vi "OPCUAServer.vi"() -> ()   [LabVIEW 2018]
uses:
  <vilib>/OPCUA/server/Read Double.vi
  <vilib>/OPCUA/NI OPC UA Server.lvlib
panel:
  in  "Tab Control":enum32{"OPC", "SQL Server", "Error Handler"}(tab)
  out "Temperature [C]":dbl=25.00772115553251 format="%.2g"
  out "Server Endpoint URL":string="opc.tcp://XPS15HPH:49580"
  out "Item Node Id":string="ns=2;s=ProcessData.Temperature"
  in  "Write to SQL Server":bool
  in  "Database Connection":T1={"Data Source Name"="XPS15HPH\\SQLEXPRESS", "Database Name"="MEASUREMENTS", "User Name"="sa", "Password"="ullabella"}
  out "Error Message":errorcluster
  out "Status":bool
  out "Current Time":string="2018-10-12 13:39:17"
  out "Error Out":errorcluster
  in  "Error In":errorcluster
  in  "Stop OPC Server":bool
  in  "Start OPC Server":bool
  in  "Exit Button":bool
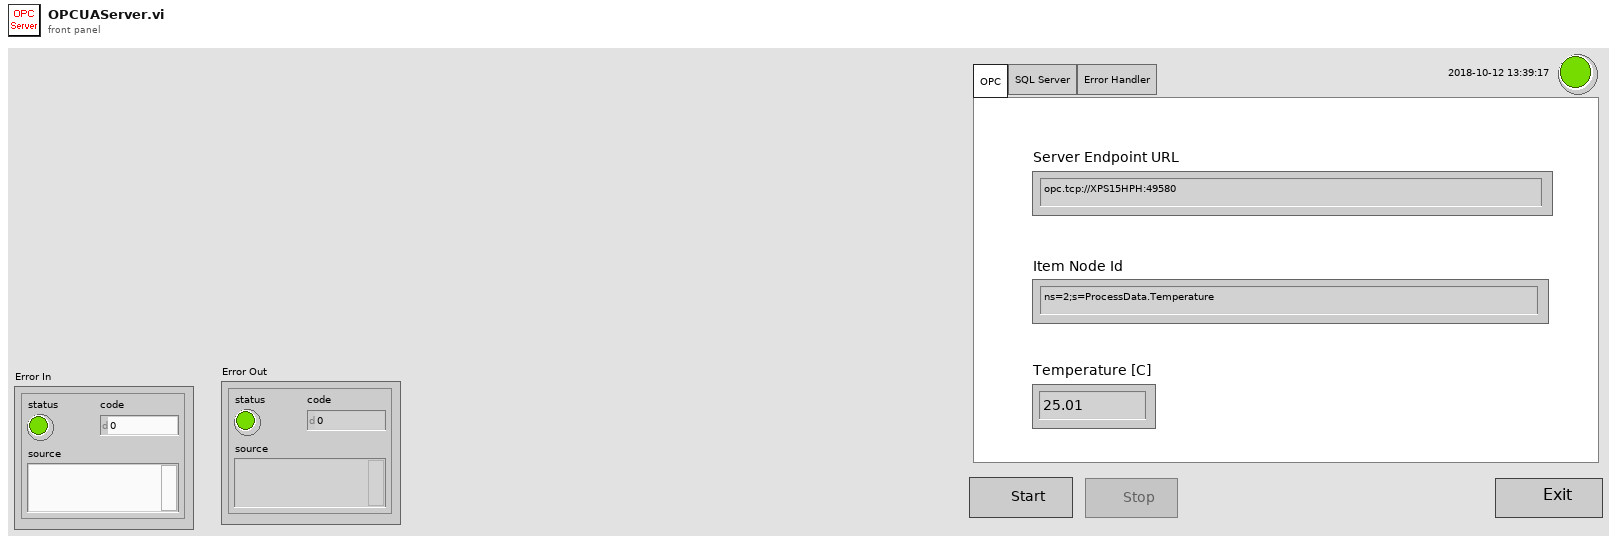
[diagram p1: front panel]
types:
  T1 = cluster{"Data Source Name":string, "Database Name":string, "User Name":string, "Password":string}
  T2 = enum8{"Enabled", "Disabled", "Disabled and Grayed Out"}
  T3 = cluster{"name":string, "data type":u16, "access level":u16, "description":string}
  T4 = typedef "OPC UA Server Refnum.ctl" = refnum<k21>
  T5 = typedef "NodeId.ctl" = string
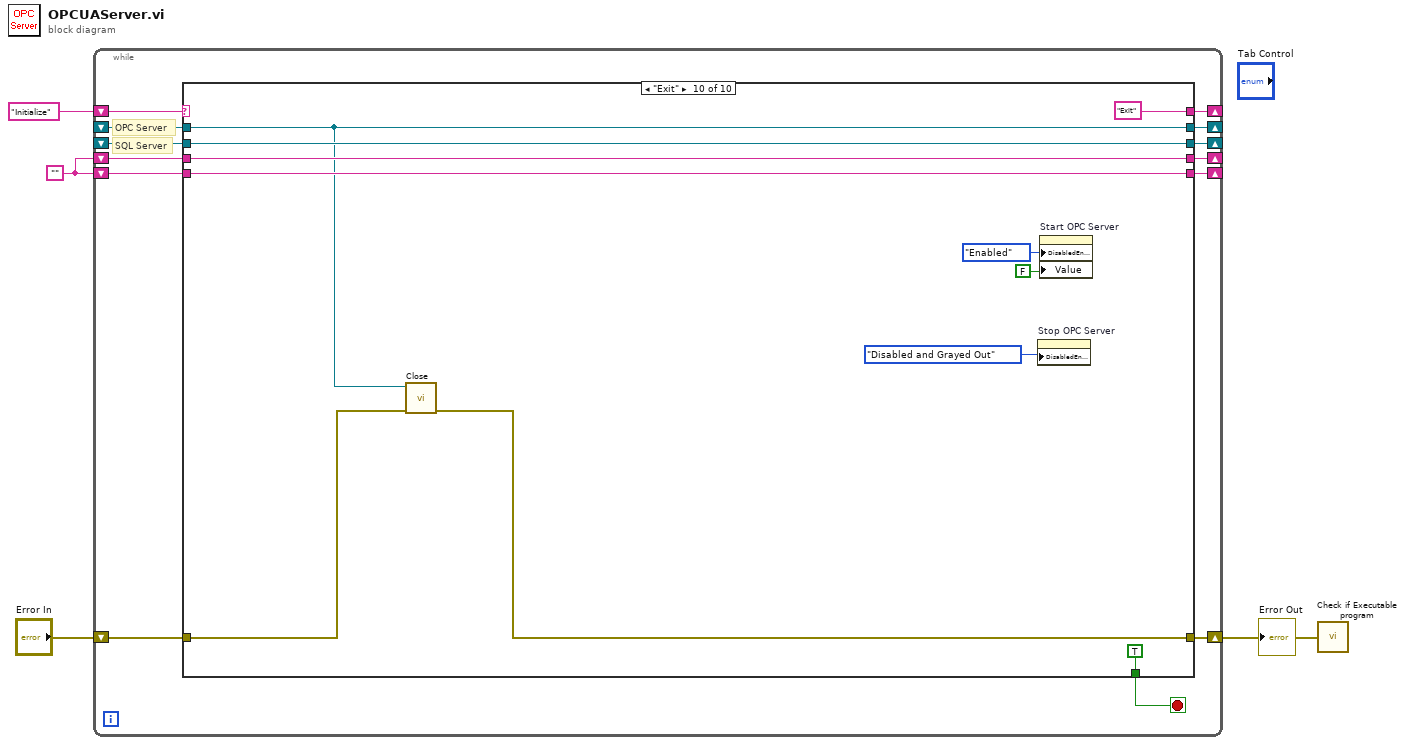
[diagram p0: block diagram]
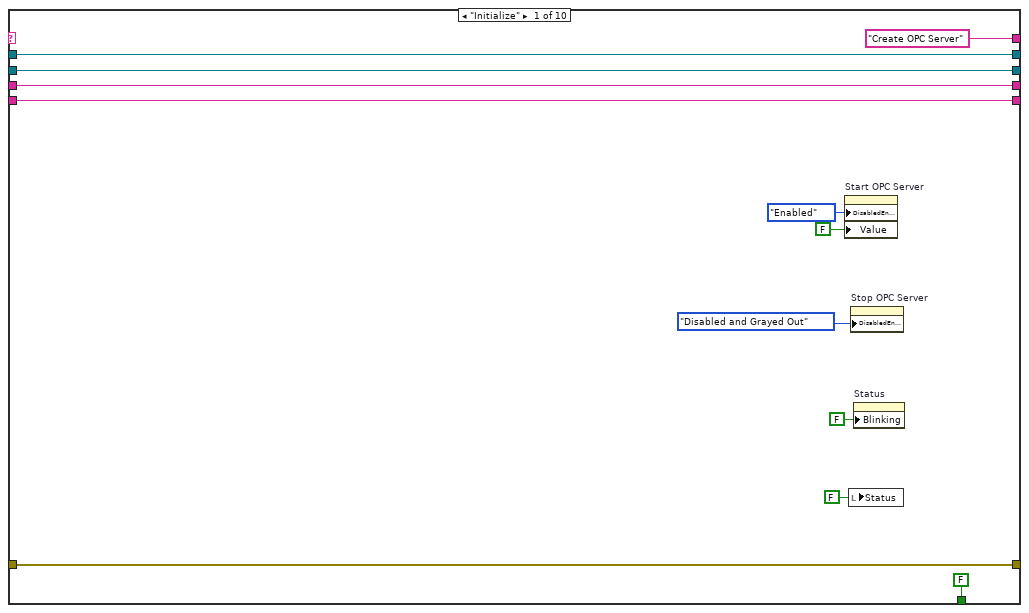
[diagram p2: hidden frame]
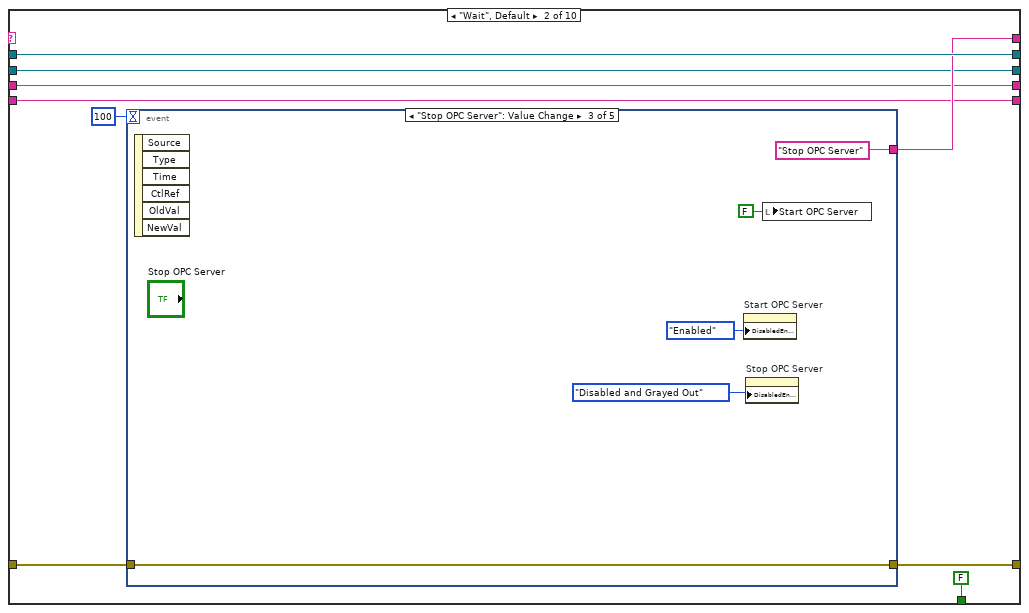
[diagram p3: hidden frame]
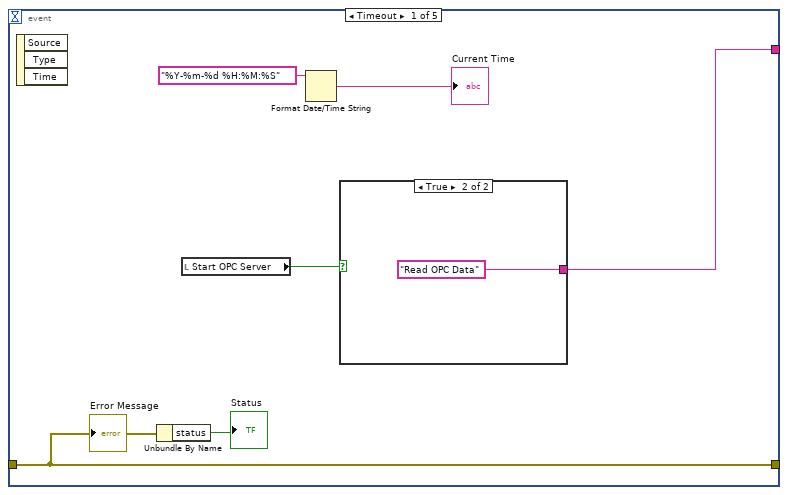
[diagram p4: hidden frame]
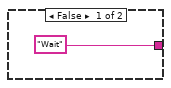
[diagram p5: hidden frame]
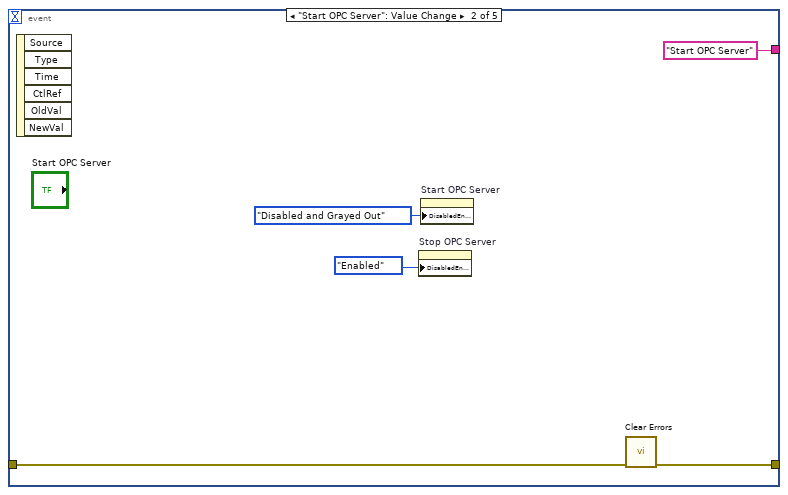
[diagram p6: hidden frame]
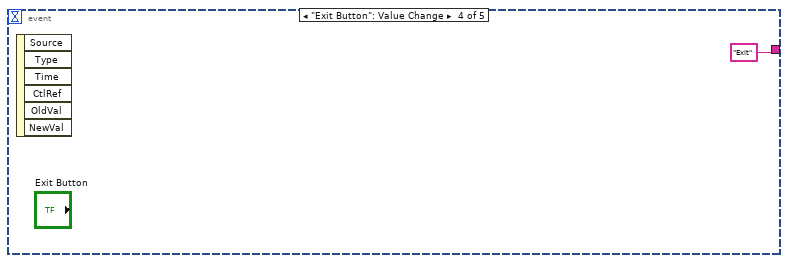
[diagram p7: hidden frame]
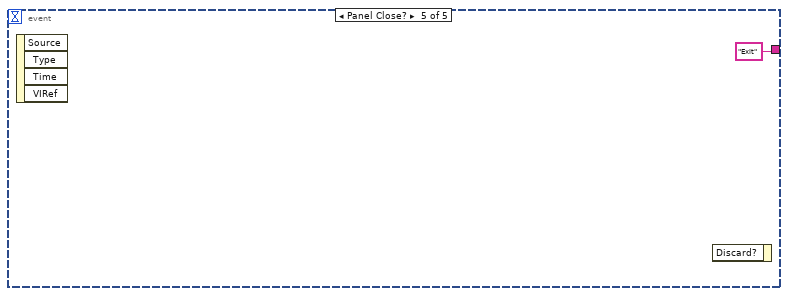
[diagram p8: hidden frame]
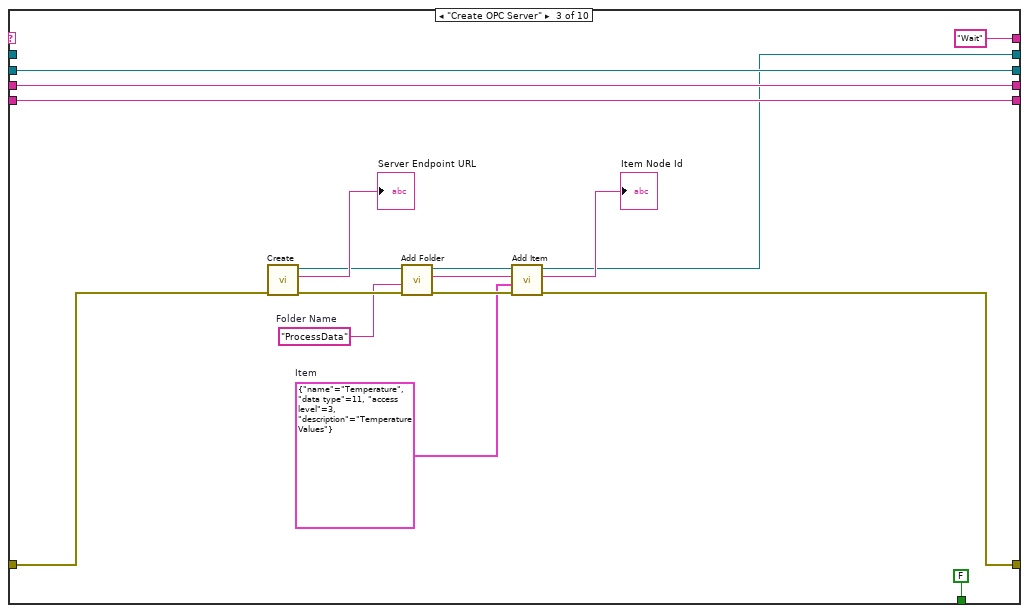
[diagram p9: hidden frame]
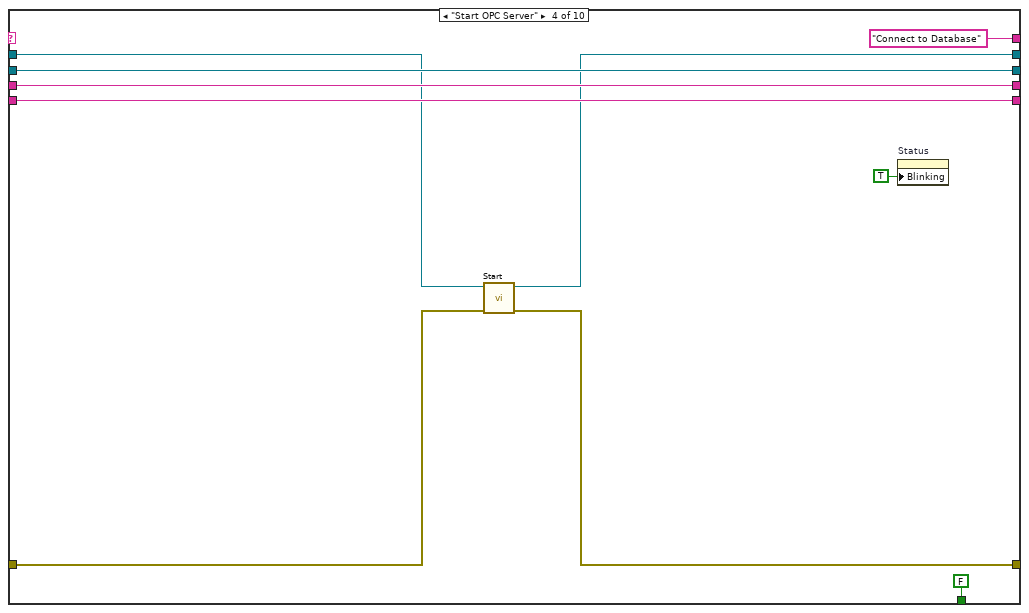
[diagram p10: hidden frame]
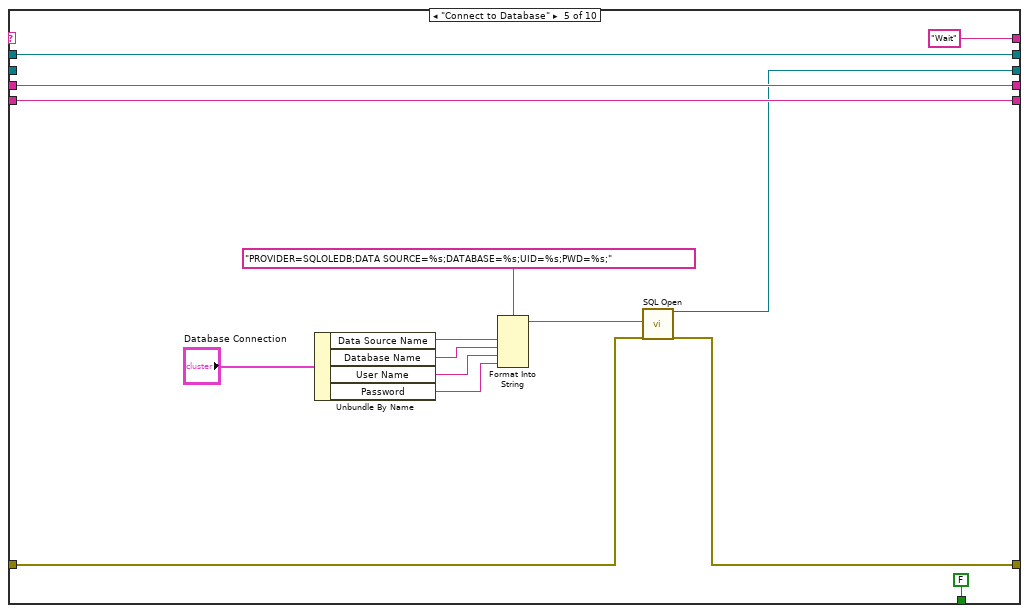
[diagram p11: hidden frame]
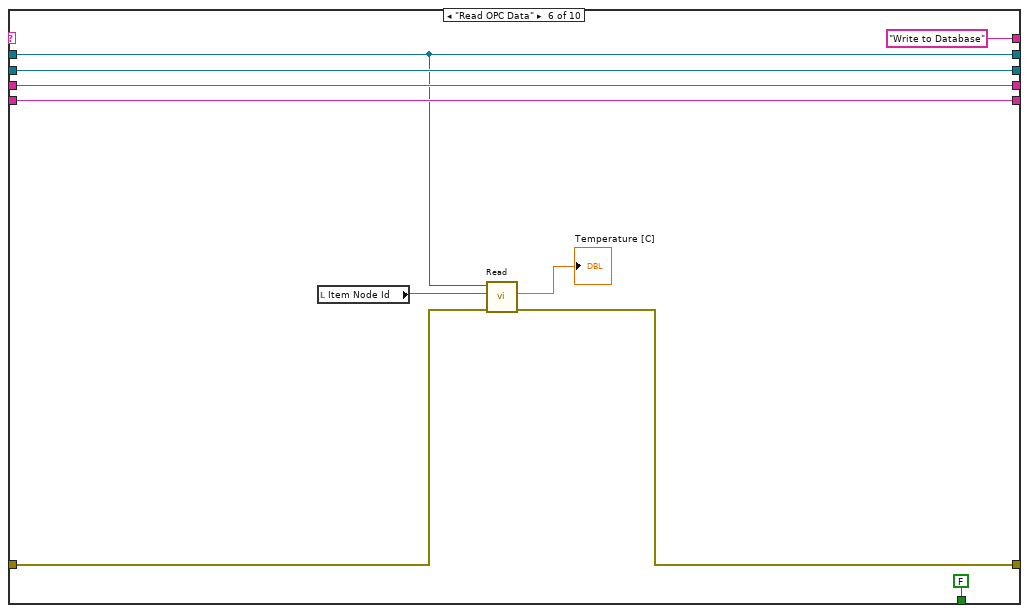
[diagram p12: hidden frame]
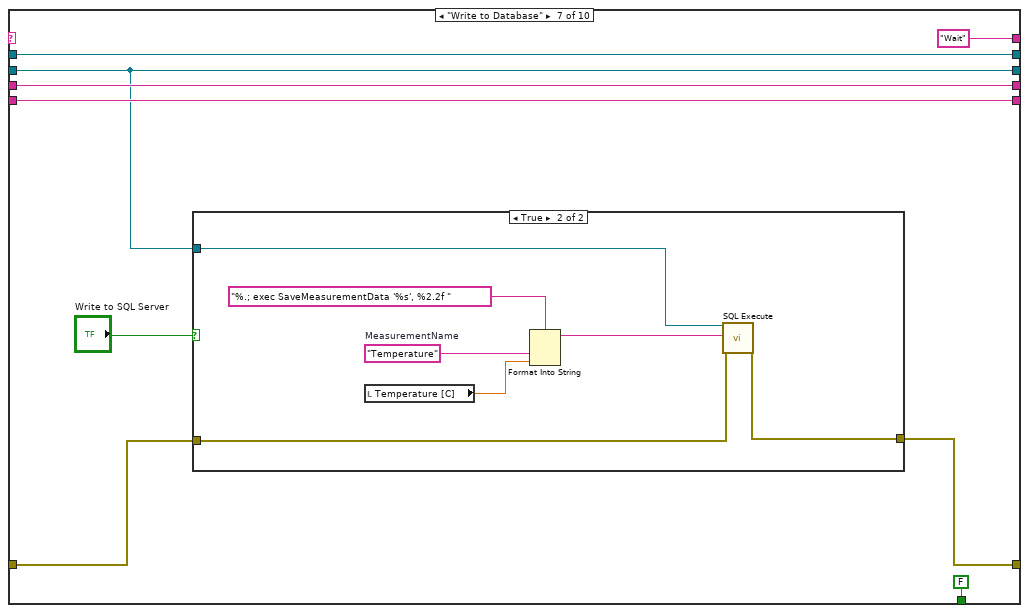
[diagram p13: hidden frame]
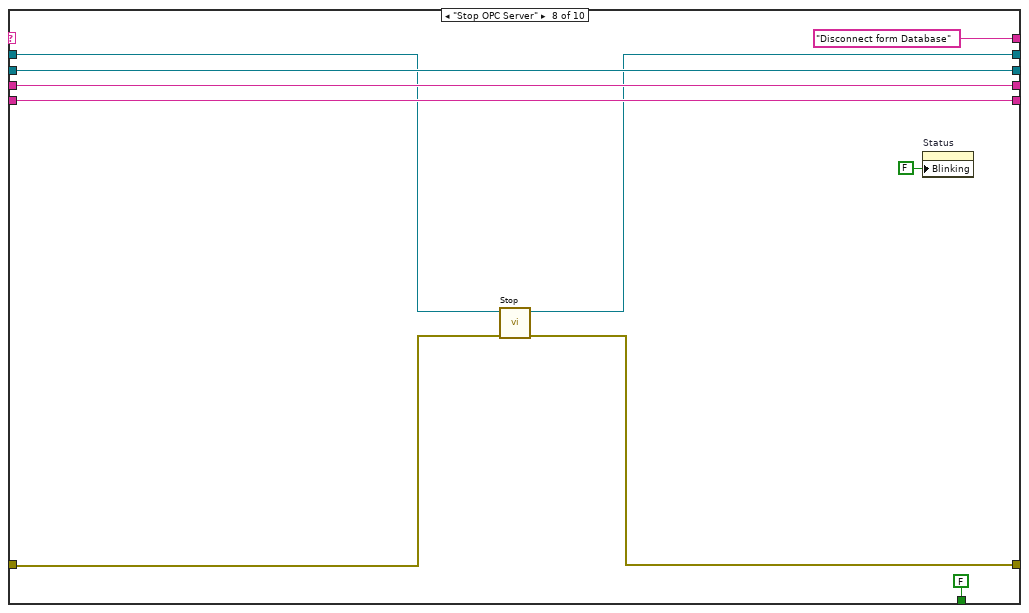
[diagram p15: hidden frame]
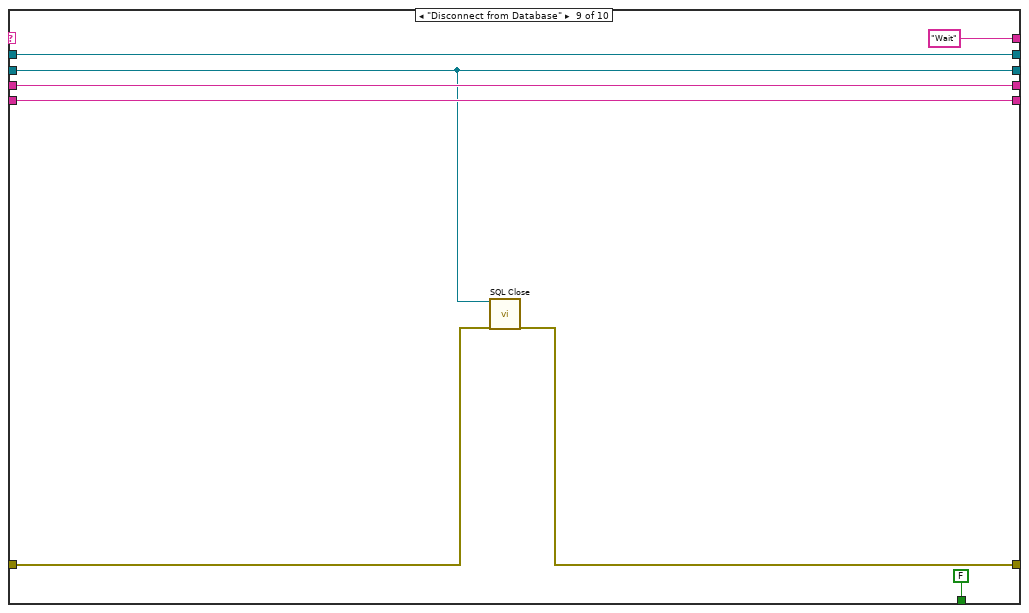
[diagram p16: hidden frame]
diagram:
  w2 = ""
  n1 = while {
    shift-right: [w16] -> _
    shift-left: "Initialize" -> [w17]
    shift-right: [w14] -> _
    shift-left: _ -> [w15]
    shift-right: [w11] -> _
    shift-left: _ -> [w12]
    shift-right: [w9] -> _
    shift-left: w2 -> [w10]
    shift-right: [w7] -> _
    shift-left: w2 -> [w8]
    shift-right: [w5] -> w1
    shift-left: "Error In" -> [w6]
    stop <- w13 stop-if-true
    # "SQL Server"
    # "OPC Server"
    n2 = case shown="\"Exit\"" w17 {
      tunnel: ["Create OPC Server" w36 "Wait" "Connect to Database" "Wait" "Write to Database" "Wait" "Disconnect form Database" "Wait" "Exit"] -> w16
      tunnel: w15 -> [w28 w37 _ w77 w100 w105 w119 w131 w145 w148]
      tunnel: [w28 w37 w60 w78 w100 w105 w119 w132 w145 w148] -> w14
      tunnel: [FALSE FALSE FALSE FALSE FALSE FALSE FALSE FALSE FALSE TRUE] -> w13
      tunnel: w12 -> [w26 w34 w71 w84 _ w109 w111 w133 w138 w155]
      tunnel: [w26 w34 w71 w84 w86 w109 w111 w133 w138 w155] -> w11
      tunnel: w10 -> [w25 w33 w74 w83 w98 w108 w116 w136 w143 w154]
      tunnel: [w25 w33 w74 w83 w98 w108 w116 w136 w143 w154] -> w9
      tunnel: w8 -> [w24 w32 w73 w82 w97 w107 w115 w135 w142 w153]
      tunnel: [w24 w32 w73 w82 w97 w107 w115 w135 w142 w153] -> w7
      tunnel: w6 -> [w23 w30 w61 w79 w95 w103 w114 w130 w140 w146]
      tunnel: [w23 w31 w59 w80 w94 w104 w113 w129 w139 w147] -> w5
      frame "Initialize" {
        n3 = property on="Start OPC Server" class="Bool (strict)"("DisabledEnum"=T2."Enabled" ("Disabled"), "Value"=FALSE ("Start DAQ Button")) -> ()  [unwired: 2 in, 2 out]
        n4 = local write "Status"(FALSE ("Status")) -> ()
        n5 = property on="Stop OPC Server" class="Bool"("DisabledEnum"=T2."Disabled and Grayed Out" ("Disabled")) -> ()  [unwired: 2 in, 2 out]
        n6 = property on="Status" class="Bool (strict)"("Blinking"=FALSE) -> ()  [unwired: 2 in, 2 out]
      }
      frame "Wait", Default {
        n7 = event shown="[2] \"Stop OPC Server\": Value Change" {
          selector: _ -> [_ _ _ _ _]
          dyn-events: _ -> [_ _ _ _ _]
          timeout: 100 -> [_ _ _ _ _]
          tunnel: [w41 "Start OPC Server" "Stop OPC Server" "Exit" "Exit"] -> w36
          tunnel: w30 -> [w39 w48 w56 _ _]
          tunnel: [w39 w47 w56 _ _] -> w31
          event Timeout {
            n8 = event-data() -> ()  [unwired: 1 in, 3 out]
            n9 = Unbundle By Name(w39) -> ("status"=→"Status":bool)
            n10 = local read "Start OPC Server"() -> (w42:bool)
            n11 = Format Date/Time String(time format string (%c)="%Y-%m-%d %H:%M:%S") -> (date/time string=→"Current Time":string)  [unwired: 2 in]
            n12 = case shown="True" w42 {
              tunnel: ["Wait" "Read OPC Data"] -> w41
              frame False {
              }
              frame True {
              }
            }
            "Error Message" <- w39
          }
          event "Start OPC Server": Value Change {
            n13 = event-data() -> ()  [unwired: 1 in, 6 out]
            n14 = property on="Stop OPC Server" class="Bool"("DisabledEnum"=T2."Enabled" ("Disabled")) -> ()  [unwired: 2 in, 2 out]
            n15 = property on="Start OPC Server" class="Bool (strict)"("DisabledEnum"=T2."Disabled and Grayed Out" ("Disabled")) -> ()  [unwired: 2 in, 2 out]
            n16 = call <vilib>:"Clear Errors.vi"("error in (no error)"=w48) -> ("error out"=w47:errorcluster)  [unwired: 5 in, 1 out]
          }
          event "Stop OPC Server": Value Change {
            n17 = event-data() -> ()  [unwired: 1 in, 6 out]
            n18 = property on="Start OPC Server" class="Bool (strict)"("DisabledEnum"=T2."Enabled" ("Disabled")) -> ()  [unwired: 2 in, 2 out]
            n19 = property on="Stop OPC Server" class="Bool"("DisabledEnum"=T2."Disabled and Grayed Out" ("Disabled")) -> ()  [unwired: 2 in, 2 out]
            n20 = local write "Start OPC Server"(FALSE ("Start OPC Server")) -> ()
          }
          event "Exit Button": Value Change {
            n21 = event-data() -> ()  [unwired: 1 in, 6 out]
          }
          event Panel Close? {
            n22 = event-data() -> ()  [unwired: 1 in, 4 out]
            n23 = event-data() -> ()  [unwired: 2 in, 1 out]
          }
        }
      }
      frame "Create OPC Server" {
        w63 = T3 {"name"="Temperature", "data type"=11, "access level"=3, "description"="Temperature Values"}  # Item
        w67 = "ProcessData"  # Folder Name
        n24 = call <vilib>:"Create.vi"("error in (no error)"=w61) -> ("error out"=w70:errorcluster, "server endpoint URL"=→"Server Endpoint URL":string, "OPC UA server refnum out"=w66:T4)  [unwired: 8 in]
        n25 = call <vilib>:"Add Folder.vi"("error in (no error)"=w70, "folder name"=w67, "OPC UA server refnum in"=w66) -> ("error out"=w69:errorcluster, "folder node ID"=w64:T5, "OPC UA server refnum out"=w65:T4)  [unwired: 5 in]
        n26 = call <vilib>:"Add Item.vi"("error in (no error)"=w69, "item"=w63, "parent folder node ID"=w64, "OPC UA server refnum in"=w65) -> ("error out"=w59:errorcluster, "item node ID"=→"Item Node Id":T5, "OPC UA server refnum out"=w60:T4)  [unwired: 3 in, 1 out]
      }
      frame "Start OPC Server" {
        n27 = call <vilib>:"Start.vi"("error in (no error)"=w79, "OPC UA server refnum in"=w77) -> ("error out"=w80:errorcluster, "OPC UA server refnum out"=w78:T4)  [unwired: 7 in, 1 out]
        n28 = property on="Status" class="Bool (strict)"("Blinking"=TRUE) -> ()  [unwired: 2 in, 2 out]
      }
      frame "Connect to Database" {
        n29 = Unbundle By Name("Database Connection") -> ("Data Source Name"=w90:string, "Database Name"=w89:string, "User Name"=w88:string, "Password"=w87:string)
        n30 = Format Into String(format string="PROVIDER=SQLOLEDB;DATA SOURCE=%s;DATABASE=%s;UID=%s;PWD=%s;", w90, w89, w88, w87) -> (resulting string=w92:string)  [unwired: 2 in, 1 out]
        n31 = call <vilib>:"SQL Open.vi"("ConnectionString In"=w92, "Error in (no error)"=w95) -> ("Connection Out"=w86:refnum<k7>, "Error out"=w94:errorcluster)  [unwired: 16 in]
      }
      frame "Read OPC Data" {
        n32 = local read "Item Node Id"() -> (w102:string)
        n33 = call-poly <vilib>:"Read.vi"("error in (no error)"=w103, "node ID"=w102, "OPC UA server refnum in"=w105) -> ("error out"=w104:errorcluster, "value"=→"Temperature [C]":dbl)  [unwired: 4 in, 3 out]
      }
      frame "Write to Database" {
        n34 = case shown="True" "Write to SQL Server" {
          tunnel: w114 -> [w120 w123]
          tunnel: [w120 w122] -> w113
          tunnel: w111 -> [_ w121]
          frame False {
          }
          frame True {
            w125 = "Temperature"  # MeasurementName
            n35 = local read "Temperature [C]"() -> (w124:dbl)
            n36 = Format Into String "Format Into String"(format string="%.; exec SaveMeasurementData '%s', %2.2f ", w125, w124) -> (resulting string=w126:string)  [unwired: 2 in, 1 out]
            n37 = call <vilib>:"SQL Execute.vi"("Connection In"=w121, "SQL Query"=w126, "Error in (no error)"=w123) -> ("Error out"=w122:errorcluster)  [unwired: 15 in, 1 out]
          }
        }
      }
      frame "Stop OPC Server" {
        n38 = call <vilib>:"Stop.vi"("error in (no error)"=w130, "OPC UA server refnum in"=w131) -> ("error out"=w129:errorcluster, "OPC UA server refnum out"=w132:T4)  [unwired: 8 in]
        n39 = property on="Status" class="Bool (strict)"("Blinking"=FALSE) -> ()  [unwired: 2 in, 2 out]
      }
      frame "Disconnect from Database" {
        n40 = call <vilib>:"SQL Close.vi"("Connection In"=w138, "Error in (no error)"=w140) -> ("Error out"=w139:errorcluster)  [unwired: 17 in]
      }
      frame "Exit" {
        n41 = call <vilib>:"Close.vi"("error in (no error)"=w146, "OPC UA server refnum in"=w148) -> ("error out"=w147:errorcluster)  [unwired: 9 in]
        n42 = property on="Stop OPC Server" class="Bool"("DisabledEnum"=T2."Disabled and Grayed Out" ("Disabled")) -> ()  [unwired: 2 in, 2 out]
        n43 = property on="Start OPC Server" class="Bool (strict)"("DisabledEnum"=T2."Enabled" ("Disabled"), "Value"=FALSE ("Start DAQ Button")) -> ()  [unwired: 2 in, 2 out]
      }
    }
  }
  "Error Out" <- w1
  n44 = call "Check if Executable program.vi"("error in (no error)"=w1) -> ()  [unwired: 1 out]
